vi "sub.vi"(11 "Waveform Graph 8":waveform(dbl)(graph)) -> (0 "appended array":bool[](array[boolean]))   [LabVIEW 2019]
panel:
  out "error out":errorcluster
  in  "error in (no error)":errorcluster
  out "1209 Hz":dynamicdata(graph) caption="Filtered Signal"
  out "1336 Hz":dynamicdata(graph) caption="Filtered Signal"
  out "1477 Hz":dynamicdata(graph) caption="Filtered Signal"
  out "852 Hz":dynamicdata(graph) caption="Filtered Signal"
  out "770 Hz":dynamicdata(graph) caption="Filtered Signal"
  out "941 Hz":dynamicdata(graph) caption="Filtered Signal"
  out "697 Hz":dynamicdata(graph) caption="Filtered Signal"
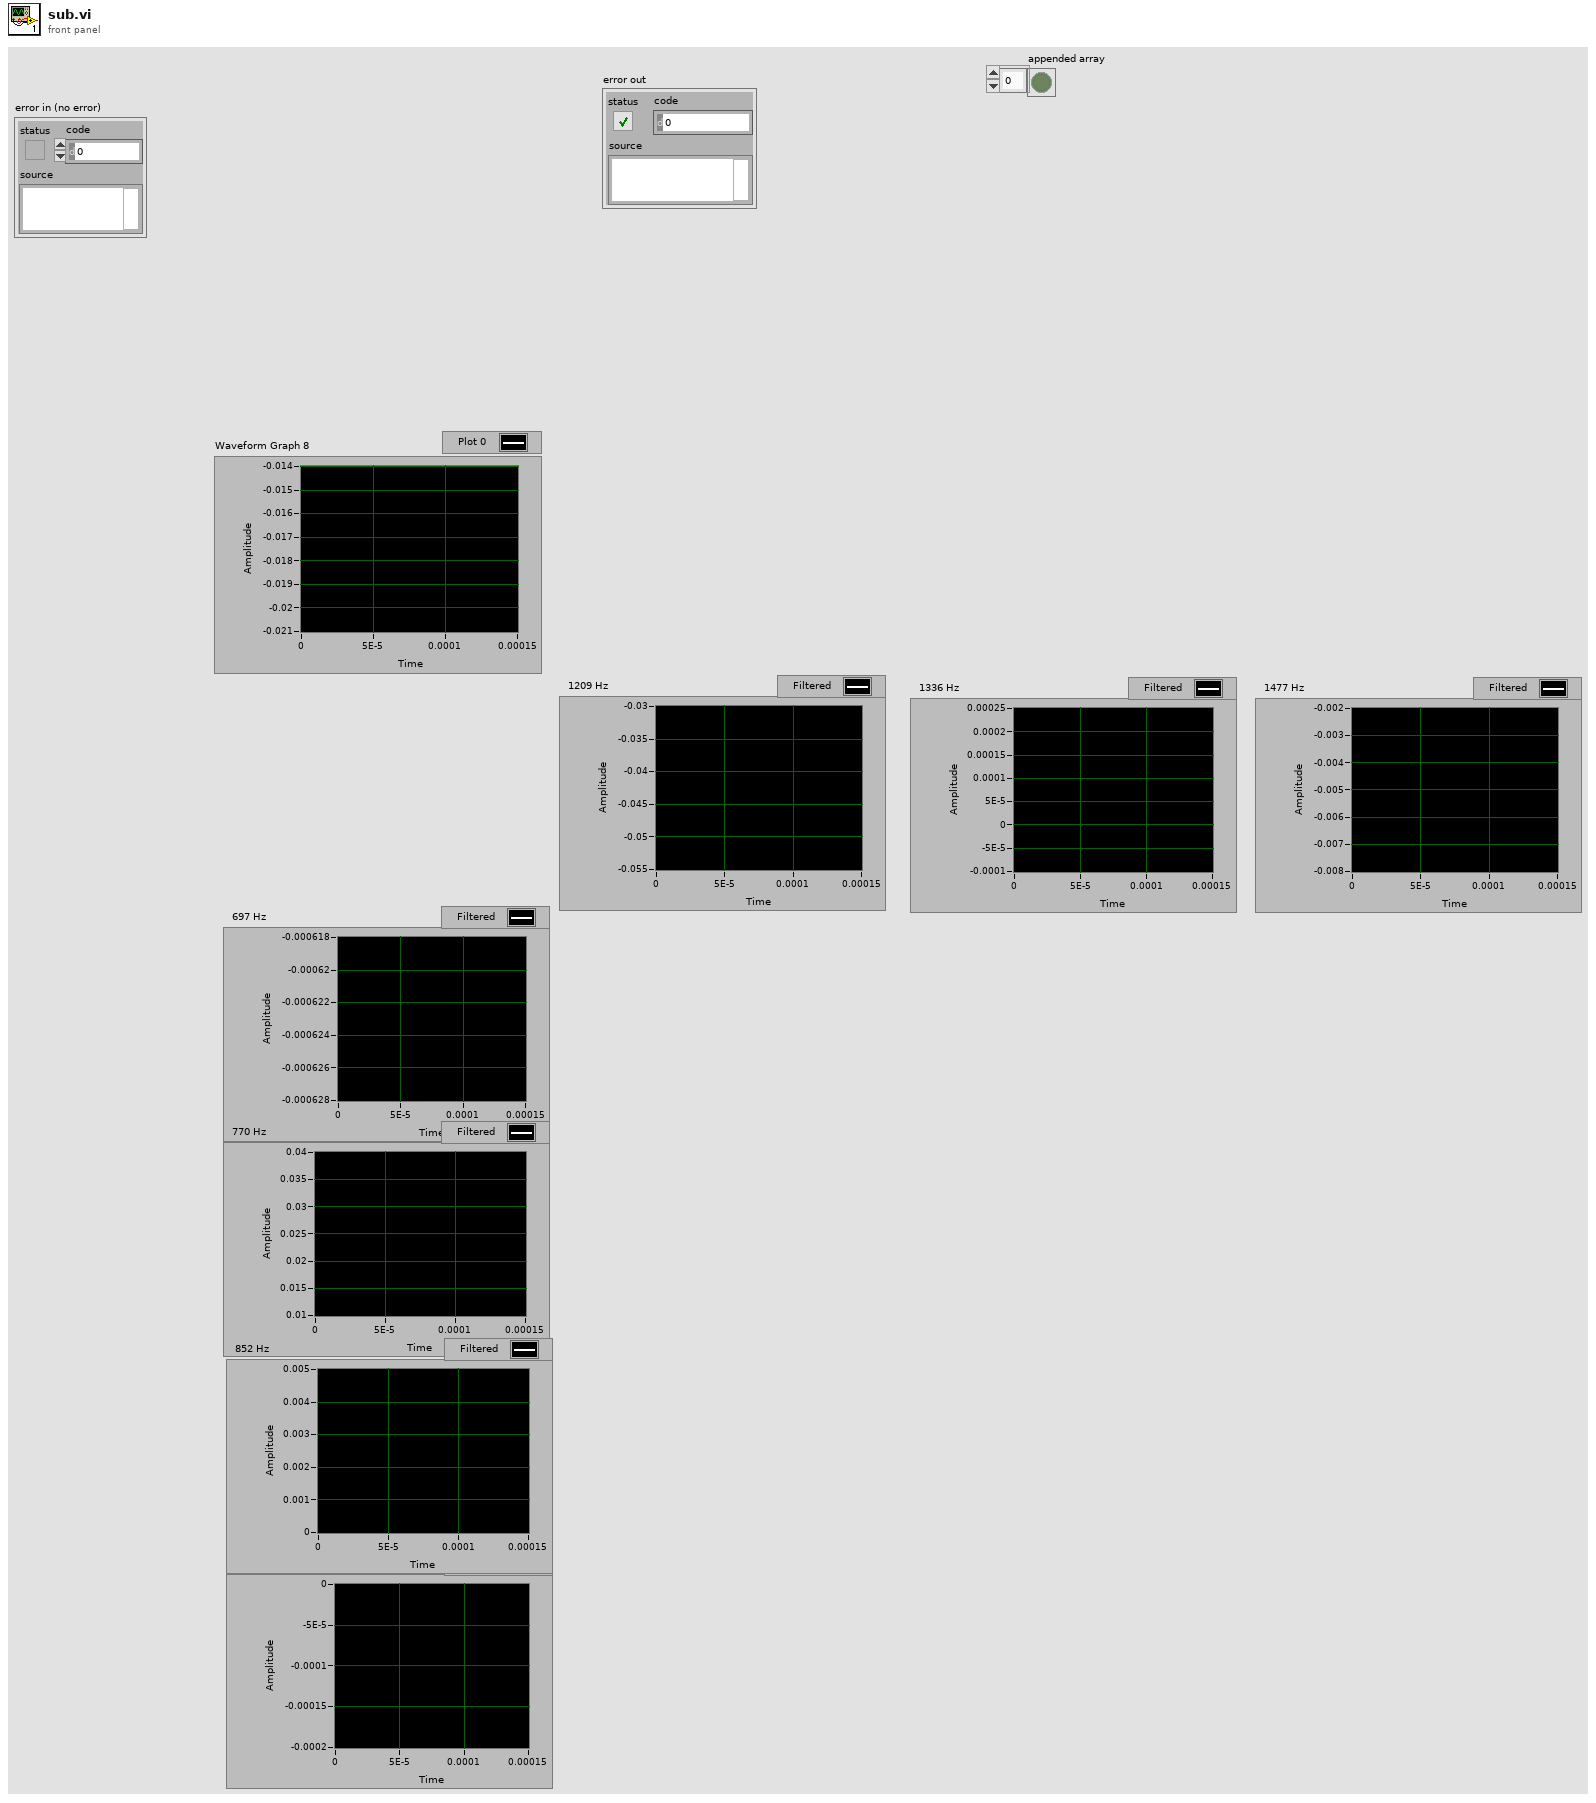
[diagram p1: front panel]
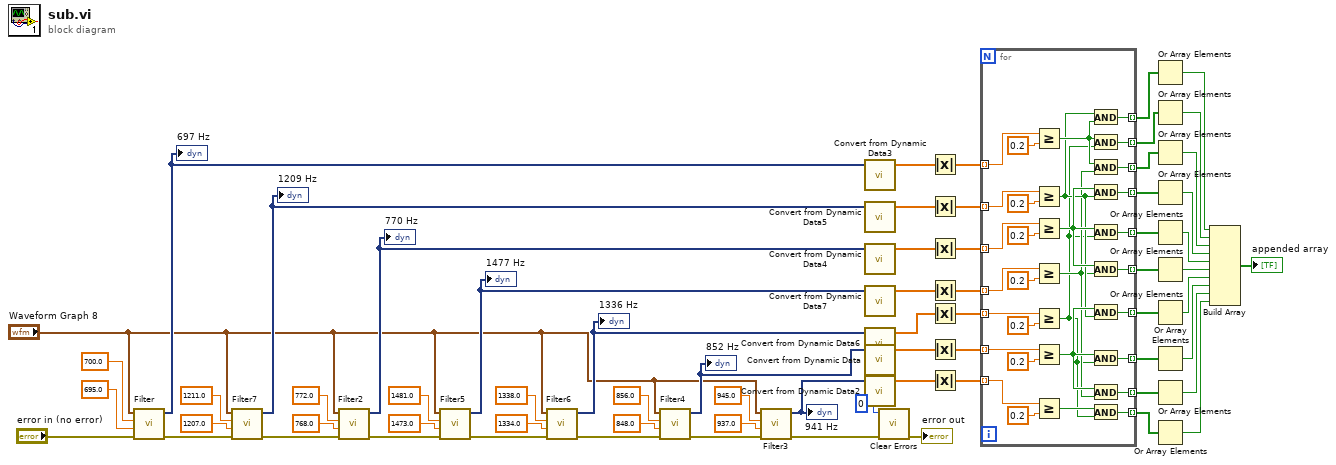
[diagram p0: block diagram]
diagram:
  n1 = call "Filter"("error in (no error)"="error in (no error)", "Lower Cut-Off"=695.0, "Upper Cut-Off"=700.0, "Signal"="Waveform Graph 8") -> ("error out"=w44:errorcluster, "Filtered Signal"=w59:dynamicdata)  [unwired: 6 in]
  "697 Hz" <- w59
  n2 = call "Filter7"("error in (no error)"=w44, "Lower Cut-Off"=1207.0, "Upper Cut-Off"=1211.0, "Signal"="Waveform Graph 8") -> ("error out"=w43:errorcluster, "Filtered Signal"=w51:dynamicdata)  [unwired: 6 in]
  "1209 Hz" <- w51
  n3 = call "Filter2"("error in (no error)"=w43, "Lower Cut-Off"=768.0, "Upper Cut-Off"=772.0, "Signal"="Waveform Graph 8") -> ("error out"=w42:errorcluster, "Filtered Signal"=w56:dynamicdata)  [unwired: 6 in]
  "770 Hz" <- w56
  n4 = call "Filter5"("error in (no error)"=w42, "Lower Cut-Off"=1473.0, "Upper Cut-Off"=1481.0, "Signal"="Waveform Graph 8") -> ("error out"=w41:errorcluster, "Filtered Signal"=w49:dynamicdata)  [unwired: 6 in]
  "1477 Hz" <- w49
  n5 = call "Filter6"("error in (no error)"=w41, "Lower Cut-Off"=1334.0, "Upper Cut-Off"=1338.0, "Signal"="Waveform Graph 8") -> ("error out"=w40:errorcluster, "Filtered Signal"=w50:dynamicdata)  [unwired: 6 in]
  "1336 Hz" <- w50
  n6 = call "Filter4"("error in (no error)"=w40, "Lower Cut-Off"=848.0, "Upper Cut-Off"=856.0, "Signal"="Waveform Graph 8") -> ("error out"=w39:errorcluster, "Filtered Signal"=w57:dynamicdata)  [unwired: 6 in]
  "852 Hz" <- w57
  n7 = call "Filter3"("error in (no error)"=w39, "Lower Cut-Off"=937.0, "Upper Cut-Off"=945.0, "Signal"="Waveform Graph 8") -> ("error out"=w1:errorcluster, "Filtered Signal"=w58:dynamicdata)  [unwired: 6 in]
  "941 Hz" <- w58
  n8 = call "Convert from Dynamic Data3"("Dynamic Data Type"=w59) -> ("Array"=w29:dbl[])  [unwired: 3 in]
  n9 = call "Convert from Dynamic Data5"("Dynamic Data Type"=w51) -> ("Array"=w35:dbl[])  [unwired: 3 in]
  n10 = call "Convert from Dynamic Data4"("Dynamic Data Type"=w56) -> ("Array"=w34:dbl[])  [unwired: 3 in]
  n11 = call "Convert from Dynamic Data7"("Dynamic Data Type"=w49) -> ("Array"=w33:dbl[])  [unwired: 3 in]
  n12 = call "Convert from Dynamic Data6"("Dynamic Data Type"=w50) -> ("Array"=w32:dbl[])  [unwired: 3 in]
  n13 = call "Convert from Dynamic Data"("Dynamic Data Type"=w57) -> ("Array"=w31:dbl[])  [unwired: 3 in]
  n14 = call "Convert from Dynamic Data2"("Dynamic Data Type"=w58) -> ("Array"=w30:dbl[])  [unwired: 3 in]
  n15 = call <vilib>:"Clear Errors.vi"("error in (no error)"=w1, "specific error code to clear (0: all)"=0) -> ("error out"=→"error out":errorcluster)  [unwired: 4 in, 1 out]
  n16 = Absolute Value(x=w29) -> (abs(x)=w36:dbl[])
  n17 = Absolute Value(x=w35) -> (abs(x)=w28:dbl[])
  n18 = Absolute Value(x=w34) -> (abs(x)=w27:dbl[])
  n19 = Absolute Value(x=w33) -> (abs(x)=w26:dbl[])
  n20 = Absolute Value(x=w32) -> (abs(x)=w25:dbl[])
  n21 = Absolute Value(x=w31) -> (abs(x)=w24:dbl[])
  n22 = Absolute Value(x=w30) -> (abs(x)=w23:dbl[])
  n23 = for {
    tunnel: w24 -> [w98] mode=indexing
    tunnel: w27 -> [w90] mode=indexing
    tunnel: w36 -> [w89] mode=indexing
    tunnel: w23 -> [w88] mode=indexing
    tunnel: w28 -> [w87] mode=indexing
    tunnel: w25 -> [w86] mode=indexing
    tunnel: w26 -> [w85] mode=indexing
    tunnel: [w84] -> w22 mode=indexing
    tunnel: [w83] -> w21 mode=indexing
    tunnel: [w82] -> w20 mode=indexing
    tunnel: [w79] -> w19 mode=indexing
    tunnel: [w78] -> w18 mode=indexing
    tunnel: [w77] -> w17 mode=indexing
    tunnel: [w73] -> w16 mode=indexing
    tunnel: [w72] -> w15 mode=indexing
    tunnel: [w71] -> w14 mode=indexing
    tunnel: [w68] -> w13 mode=indexing
    n24 = Greater Or Equal?(x=w89, y=0.2 ("lower limit")) -> (x >= y?=w81:bool)
    n25 = Greater Or Equal?(x=w87, y=0.2 ("lower limit")) -> (x >= y?=w75:bool)
    n26 = Greater Or Equal?(x=w90, y=0.2 ("lower limit")) -> (x >= y?=w80:bool)
    n27 = Greater Or Equal?(x=w85, y=0.2 ("lower limit")) -> (x >= y?=w74:bool)
    n28 = Greater Or Equal?(x=w86, y=0.2 ("lower limit")) -> (x >= y?=w69:bool)
    n29 = Greater Or Equal?(x=w98, y=0.2 ("lower limit")) -> (x >= y?=w76:bool)
    n30 = Greater Or Equal?(x=w88, y=0.2 ("lower limit")) -> (x >= y?=w70:bool)
    n31 = And(x=w75, y=w81) -> (x .and. y?=w84:bool)
    n32 = And(x=w81, y=w69) -> (x .and. y?=w83:bool)
    n33 = And(x=w81, y=w74) -> (x .and. y?=w82:bool)
    n34 = And(x=w80, y=w75) -> (x .and. y?=w79:bool)
    n35 = And(x=w80, y=w69) -> (x .and. y?=w78:bool)
    n36 = And(x=w80, y=w74) -> (x .and. y?=w77:bool)
    n37 = And(x=w76, y=w75) -> (x .and. y?=w73:bool)
    n38 = And(x=w76, y=w69) -> (x .and. y?=w72:bool)
    n39 = And(x=w76, y=w74) -> (x .and. y?=w71:bool)
    n40 = And(x=w70, y=w69) -> (x .and. y?=w68:bool)
  }
  n41 = Or Array Elements(Boolean array=w22) -> (logical OR=w12:bool)
  n42 = Or Array Elements(Boolean array=w21) -> (logical OR=w11:bool)
  n43 = Or Array Elements(Boolean array=w20) -> (logical OR=w10:bool)
  n44 = Or Array Elements(Boolean array=w19) -> (logical OR=w9:bool)
  n45 = Or Array Elements(Boolean array=w18) -> (logical OR=w8:bool)
  n46 = Or Array Elements(Boolean array=w17) -> (logical OR=w7:bool)
  n47 = Or Array Elements(Boolean array=w16) -> (logical OR=w6:bool)
  n48 = Or Array Elements(Boolean array=w15) -> (logical OR=w5:bool)
  n49 = Or Array Elements(Boolean array=w14) -> (logical OR=w4:bool)
  n50 = Or Array Elements(Boolean array=w13) -> (logical OR=w3:bool)
  n51 = Build Array(w12, w11, w10, w9, w8, w7, w6, w5, w4, w3) -> (→"appended array":bool[])
